vi "SetParam.vi"(8 "error in (no error)":errorcluster caption="entrée d'erreur (pas d'erreur)", 10 "RepeatedStratifiedKFold":T1={"n_splits"=5, "n_repeats"=10, "random_state"=-1} {"random_state" min=-1}, 11 "RepeatedStratifiedKFold.lvclass":refnum<class "RepeatedStratifiedKFold.lvclass">) -> (0 "error out":errorcluster caption="sortie d'erreur", 3 "RepeatedStratifiedKFold.lvclass":refnum<class "RepeatedStratifiedKFold.lvclass">)   [LabVIEW 2020, in "RepeatedStratifiedKFold.lvclass"]
doc: "Set Parameters"
uses:
  RepeatedStratifiedKFold.lvclass
  RepeatedStratifiedKFold.lvclass/RepeatedStratifiedKFold.ctl
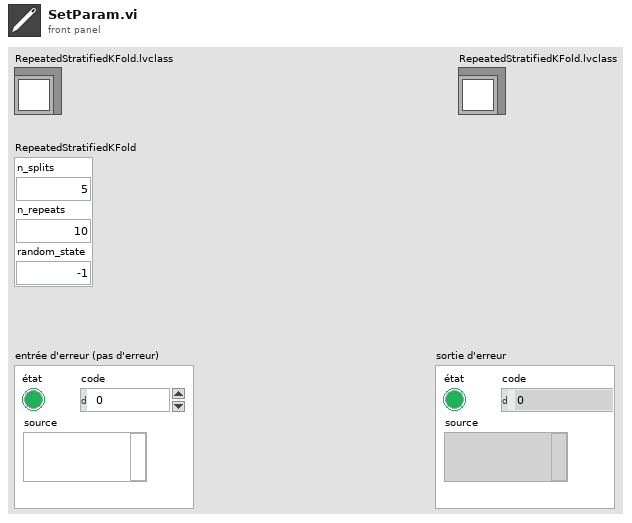
[diagram p1: front panel]
types:
  T1 = cluster{"n_splits":i32, "n_repeats":i32, "random_state":i32}
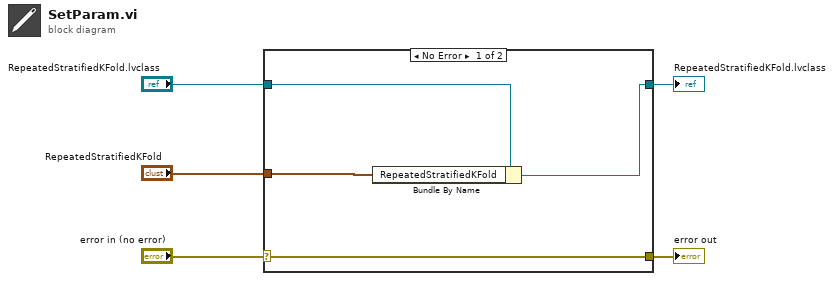
[diagram p0: block diagram]
diagram:
  n1 = case shown="No Error" "error in (no error)" {
    selector: "error in (no error)" -> [w9 w10]
    tunnel: [w9 w10] -> w4
    tunnel: [w7 w11] -> w2
    tunnel: "RepeatedStratifiedKFold.lvclass" -> [w8 w11]
    tunnel: "RepeatedStratifiedKFold" -> [w6 _]
    frame No Error {
      n2 = Bundle By Name(cluster=w8, "RepeatedStratifiedKFold"=w6) -> (w7:refnum<class "RepeatedStratifiedKFold.lvclass">)
    }
    frame Error {
    }
  }
  "error out" <- w4
  "RepeatedStratifiedKFold.lvclass" <- w2
